vi "MGCC_FntStaMach_EnableSignalCalcul.vi"(10 "Input enable 2":bool[][](array[boolean]), 11 "Input enable 1":bool[][](array[boolean])) -> ()   [LabVIEW 2016]
uses:
  MGCC_FntStaMach_gobal.vi
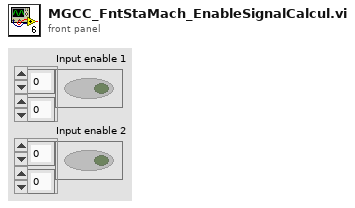
[diagram p1: front panel]
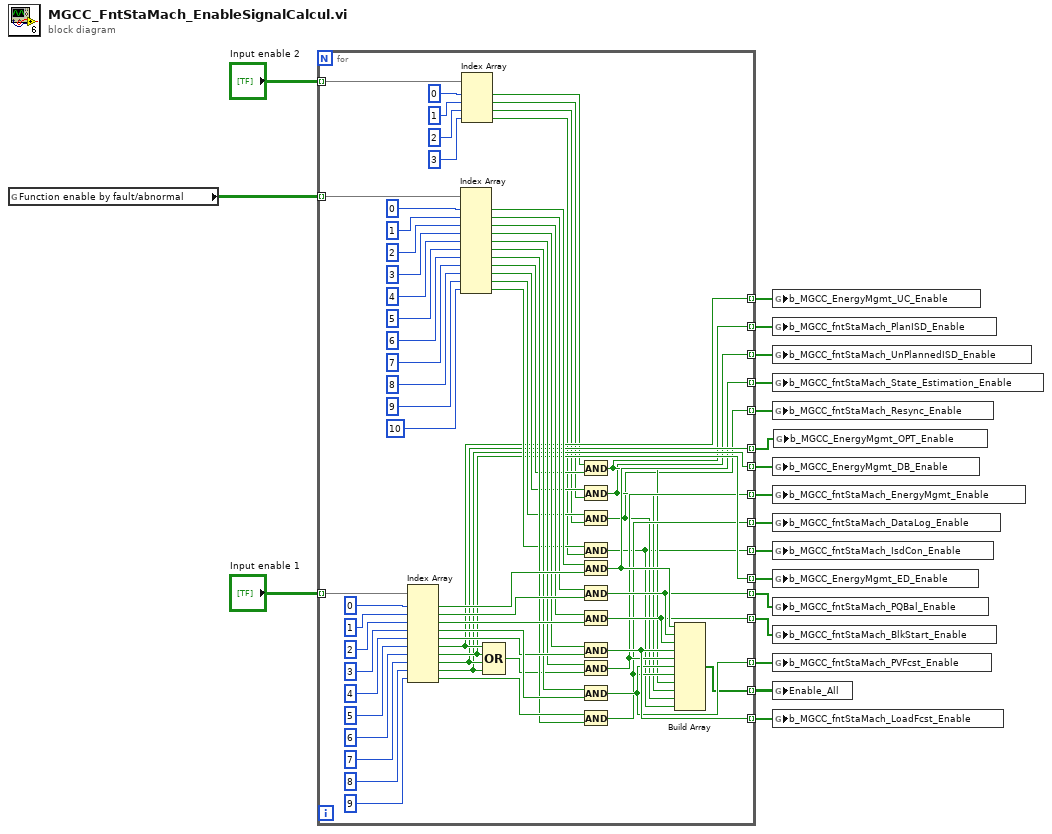
[diagram p0: block diagram]
diagram:
  n1 = global read "MGCC_FntStaMach_gobal.vi" "Function enable by fault/abnormal"() -> (w14:bool[][])
  n2 = for {
    tunnel: "Input enable 1" -> [w47] mode=indexing
    tunnel: [w46] -> w18 mode=indexing
    tunnel: [w45] -> w17 mode=indexing
    tunnel: [w44] -> w16 mode=indexing
    tunnel: [w43] -> w15 mode=indexing
    tunnel: w14 -> [w41] mode=indexing
    tunnel: [w40] -> w13 mode=indexing
    tunnel: [w39] -> w12 mode=indexing
    tunnel: [w38] -> w11 mode=indexing
    tunnel: [w37] -> w10 mode=indexing
    tunnel: [w36] -> w9 mode=indexing
    tunnel: [w35] -> w8 mode=indexing
    tunnel: [w34] -> w7 mode=indexing
    tunnel: [w33] -> w6 mode=indexing
    tunnel: [w32] -> w5 mode=indexing
    tunnel: [w31] -> w4 mode=indexing
    tunnel: [w30] -> w3 mode=indexing
    tunnel: [w29] -> w2 mode=indexing
    tunnel: "Input enable 2" -> [w28] mode=indexing
    n3 = Index Array(array=w47, index #1=0 ("index"), index #2=1 ("index"), index #3=2 ("index"), index #4=3 ("index"), index #5=4 ("index"), index #6=5 ("index"), index #7=6 ("index"), index #8=7 ("index"), index #9=8 ("index"), index #10=9 ("index")) -> (element #1=w72:bool, element #2=w75:bool, element #3=w74:bool, element #4=w71:bool, element #5=w70:bool, element #6=w46:bool, element #7=w45:bool, element #8=w44:bool, element #9=w43:bool, element #10=w73:bool)
    n4 = Index Array(array=w41, index #1=0 ("index"), index #2=1 ("index"), index #3=2 ("index"), index #4=3 ("index"), index #5=4 ("index"), index #6=5 ("index"), index #7=6 ("index"), index #8=7 ("index"), index #9=8 ("index"), index #10=9 ("index"), index #11=10 ("index")) -> (element #1=w58:bool, element #2=w57:bool, element #3=w56:bool, element #4=w55:bool, element #5=w54:bool, element #6=w53:bool, element #7=w52:bool, element #8=w51:bool, element #9=w50:bool, element #10=w49:bool, element #11=w48:bool)
    n5 = Index Array(array=w28, index #1=0 ("index"), index #2=1 ("index"), index #3=2 ("index"), index #4=3 ("index")) -> (element #1=w20:bool, element #2=w21:bool, element #3=w22:bool, element #4=w23:bool)
    n6 = Compound Arithmetic op=OR(w46, w45, w44, w43) -> (w42:bool)
    n7 = And(x=w20, y=w51) -> (x .and. y?=w33:bool)
    n8 = And(x=w50, y=w21) -> (x .and. y?=w32:bool)
    n9 = And(x=w49, y=w22) -> (x .and. y?=w31:bool)
    n10 = And(x=w48, y=w23) -> (x .and. y?=w30:bool)
    n11 = And(x=w58, y=w72) -> (x .and. y?=w40:bool)
    n12 = And(x=w57, y=w75) -> (x .and. y?=w39:bool)
    n13 = And(x=w56, y=w74) -> (x .and. y?=w38:bool)
    n14 = And(x=w55, y=w70) -> (x .and. y?=w37:bool)
    n15 = And(x=w54, y=w42) -> (x .and. y?=w36:bool)
    n16 = And(x=w53, y=w71) -> (x .and. y?=w35:bool)
    n17 = And(x=w73, y=w52) -> (x .and. y?=w34:bool)
    n18 = Build Array(w40, w39, w38, w37, w36, w35, w34, w33, w32, w31, w30) -> (w29:bool[])
  }
  n19 = global write "MGCC_FntStaMach_gobal.vi" "b_MGCC_EnergyMgmt_UC_Enable"(w18) -> ()
  n20 = global write "MGCC_FntStaMach_gobal.vi" "b_MGCC_fntStaMach_PlanISD_Enable"(w6) -> ()
  n21 = global write "MGCC_FntStaMach_gobal.vi" "b_MGCC_fntStaMach_UnPlannedISD_Enable"(w5) -> ()
  n22 = global write "MGCC_FntStaMach_gobal.vi" "b_MGCC_fntStaMach_State_Estimation_Enable"(w13) -> ()
  n23 = global write "MGCC_FntStaMach_gobal.vi" "b_MGCC_fntStaMach_Resync_Enable"(w4) -> ()
  n24 = global write "MGCC_FntStaMach_gobal.vi" "b_MGCC_EnergyMgmt_DB_Enable"(w15) -> ()
  n25 = global write "MGCC_FntStaMach_gobal.vi" "b_MGCC_fntStaMach_EnergyMgmt_Enable"(w9) -> ()
  n26 = global write "MGCC_FntStaMach_gobal.vi" "b_MGCC_fntStaMach_DataLog_Enable"(w7) -> ()
  n27 = global write "MGCC_FntStaMach_gobal.vi" "b_MGCC_fntStaMach_IsdCon_Enable"(w3) -> ()
  n28 = global write "MGCC_FntStaMach_gobal.vi" "b_MGCC_EnergyMgmt_ED_Enable"(w17) -> ()
  n29 = global write "MGCC_FntStaMach_gobal.vi" "b_MGCC_fntStaMach_PQBal_Enable"(w12) -> ()
  n30 = global write "MGCC_FntStaMach_gobal.vi" "b_MGCC_fntStaMach_BlkStart_Enable"(w11) -> ()
  n31 = global write "MGCC_FntStaMach_gobal.vi" "b_MGCC_fntStaMach_PVFcst_Enable"(w8) -> ()
  n32 = global write "MGCC_FntStaMach_gobal.vi" "Enable_All"(w2) -> ()
  n33 = global write "MGCC_FntStaMach_gobal.vi" "b_MGCC_fntStaMach_LoadFcst_Enable"(w10) -> ()
  n34 = global write "MGCC_FntStaMach_gobal.vi" "b_MGCC_EnergyMgmt_OPT_Enable"(w16) -> ()
